vi "LCB Open.vi"(8 "error in (no error)":errorcluster caption="Fehler (Eingang, kein Fehler)", 10 "PluginSearchPath":string, 11 "Device Configuration Path":string) -> (0 "error out":errorcluster caption="Fehler (Ausgang)")   [LabVIEW 2023, in "labbCAN_Bus_API.lvlib"]
doc: "LCB_Func long __stdcall LCB_Open(const char* pDeviceConfigPath);"
uses:
  labbCAN_Bus_API.lvlib
  labbCAN_Bus_API.dll
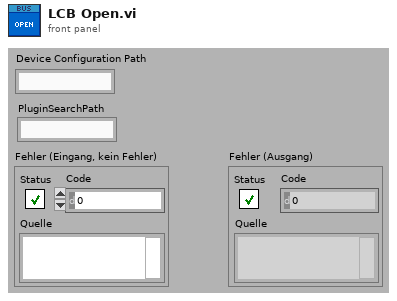
[diagram p1: front panel]
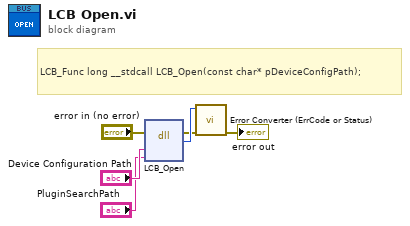
[diagram p0: block diagram]
diagram:
  # "LCB_Func long __stdcall LCB_Open(const char* pDeviceConfigPath);"
  n1 = dll-call lib="C:/GIT/DensityGradientProject/CETONI_SDK/labbCAN_Bus_API.*" fn="LCB_Open"(error in="error in (no error)", "pDeviceConfigPath"="Device Configuration Path", "PluginSearchPath"="PluginSearchPath") -> (error out=w3:errorcluster, "Rückgabetyp"=w4:i32)  [unwired: 4 in, 1 out]
  n2 = call "Error Converter (ErrCode or Status).vi"("error in (no error)"=w3, "error code"=w4) -> ("error out"=→"error out":errorcluster)  [unwired: 9 in]
